vi "Turret.vi"(5 "turret":T1, 7 "top view":T1, 9 "angle":dbl, 11 "Refnum in":T1) -> (3 "Refnum out":T1)   [LabVIEW 2018]
uses:
  <vilib>/vision/Image Controls.llb/IMAQ Image.ctl
  <vilib>/vision/NI_Vision_Development_Module.lvlib
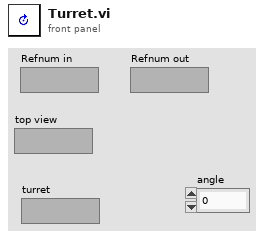
[diagram p1: front panel]
types:
  T1 = typedef "IMAQ Image.ctl" = refnum<image>
  T2 = cluster{"Blue or Luma":u8, "Green or Sat Plane":u8, "Red or Hue Plane":u8, "Alpha":u8}
  T3 = cluster{"Desired Font (Application)":enum16{"User-specified Font", "Application Font", "System Font", "Dialog Font"}, "[User-specified Font]":cluster{"Font Name":string, "Size":i16, "Strikeout?":bool, "Italic?":bool, "Underline?":bool, "Outline?":bool, "Shadow?":bool, "Bold?":bool, "Rotation Angle":dbl}, "Horizontal Alignment":i16, "Vertical Alignment":i16}
  T4 = typedef "Image Type" = u32
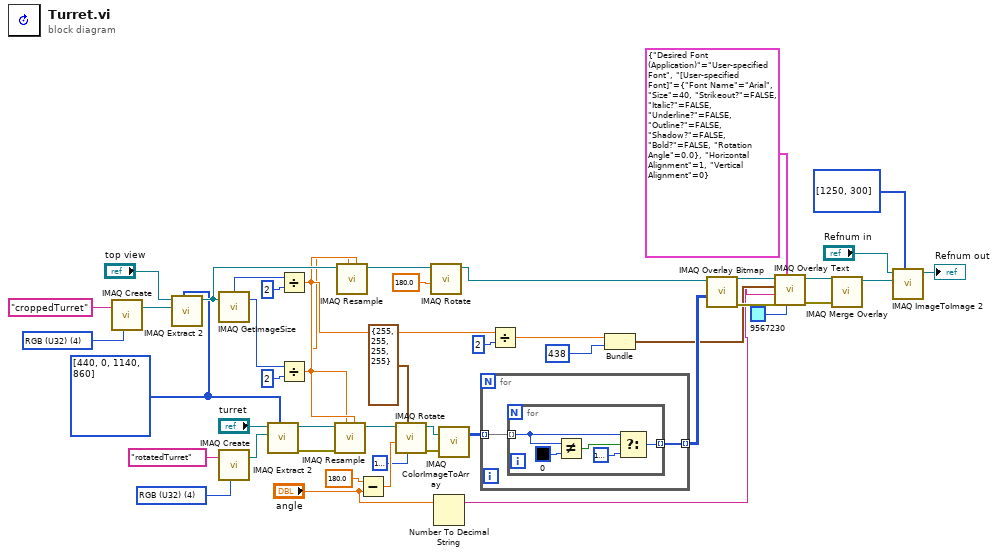
[diagram p0: block diagram]
diagram:
  w32 = T4 4 items=["Grayscale (U8)", "Grayscale (I16)", "Grayscale (SGL)", "Complex (CSG)", "RGB (U32)", "HSL (U32)", "RGB (U64)", "Grayscale (U16)"] ("Image Type")
  w40 = T4 4 items=["Grayscale (U8)", "Grayscale (I16)", "Grayscale (SGL)", "Complex (CSG)", "RGB (U32)", "HSL (U32)", "RGB (U64)", "Grayscale (U16)"] ("Image Type")
  w28 = i32[] [440, 0, 1140, 860] ("Optional Rectangle")
  n1 = call "IMAQ Create"("Image Name"="croppedTurret", "Image Type"=w40) -> ("New Image"=w41:T1)  [unwired: 3 in, 1 out]
  n2 = call "IMAQ Extract 2"("Optional Rectangle"=w28, "Image Dst"=w41, "Image Src"="top view") -> ("Image Dst Out"=w39:T1)  [unwired: 7 in, 1 out]
  n3 = call "IMAQ GetImageSize"("Image"=w39) -> ("Y Resolution"=w38:i32, "X Resolution"=w37:i32)  [unwired: 3 in, 1 out]
  n4 = call "IMAQ Create"("Image Name"="rotatedTurret", "Image Type"=w32) -> ("New Image"=w30:T1)  [unwired: 3 in, 1 out]
  n5 = call "IMAQ Extract 2"("Optional Rectangle"=w28, "Image Dst"=w30, "Image Src"="turret") -> ("error out"=w27:errorcluster, "Image Dst Out"=w26:T1)  [unwired: 7 in]
  n6 = Divide(x=w37, y=2) -> (x/y=w2:dbl)
  n7 = Divide(x=w38, y=2) -> (x/y=w1:dbl)
  n8 = call "IMAQ Resample"("X Resolution"=w2, "Y Resolution"=w1, "error in (no error)"=w27, "Image Src"=w26) -> ("Image Dst Out"=w25:T1)  [unwired: 6 in, 1 out]
  n9 = call "IMAQ Resample"("X Resolution"=w2, "Y Resolution"=w1, "Image Src"=w39) -> ("Image Dst Out"=w34:T1)  [unwired: 7 in, 1 out]
  n10 = Subtract(x=180.0 ("y"), y="angle") -> (x-y=w20:dbl)
  n11 = call "IMAQ Rotate"("Replace Value"=u32 16777216, "Color Replace Value"=T2 {"Blue or Luma"=255, "Green or Sat Plane"=255, "Red or Hue Plane"=255, "Alpha"=255}, "Angle (degrees)"=w20, "Image Src"=w25) -> ("error out"=w21:errorcluster, "Image Dst Out"=w22:T1)  [unwired: 6 in]
  n12 = call "IMAQ Rotate"("Angle (degrees)"=sgl 180.0, "Image Src"=w34) -> ("Image Dst Out"=w24:T1)  [unwired: 8 in, 1 out]
  n13 = Number To Decimal String(number="angle") -> (decimal integer string=w5:string)  [unwired: 1 in]
  n14 = call "IMAQ ColorImageToArray"("Image"=w22, "error in (no error)"=w21) -> ("Image Pixels (U32)"=w18:u32[][])  [unwired: 2 in, 2 out]
  n15 = for {
    tunnel: w18 -> [w48] mode=indexing
    tunnel: [w47] -> w17 mode=indexing
    n16 = for {
      tunnel: w48 -> [w51] mode=indexing
      tunnel: [w50] -> w47 mode=indexing
      n17 = Not Equal?(x=w51, y=u32 0) -> (x != y?=w52:bool)
      n18 = Select(t=w51, s=w52, f=u32 16777216) -> (s? t:f=w50:u32)
    }
  }
  n19 = Divide(x=w2, y=2) -> (x/y=w9:dbl)
  n20 = Bundle(w9, "y"=438) -> (w8:cluster{dbl, "y":i32})  [unwired: 1 in]
  n21 = call "IMAQ Overlay Bitmap"("Bitmap"=w17, "Image"=w24) -> ("error out"=w13:errorcluster, "Image Out"=w14:T1)  [unwired: 8 in]
  n22 = call "IMAQ Overlay Text"("Text Color (black)"=u32 9567230, "Font, Size & Style"=T3 {"Desired Font (Application)"=enum."User-specified Font", "[User-specified Font]"={"Font Name"="Arial", "Size"=40, "Strikeout?"=FALSE, "Italic?"=FALSE, "Underline?"=FALSE, "Outline?"=FALSE, "Shadow?"=FALSE, "Bold?"=FALSE, "Rotation Angle"=0.0}, "Horizontal Alignment"=1, "Vertical Alignment"=0}, "error in (no error)"=w13, "String"=w5, "Origin"=w8, "Image"=w14) -> ("error out"=w16:errorcluster, "Image Out"=w15:T1)  [unwired: 4 in]
  n23 = call "IMAQ Merge Overlay"("error in (no error)"=w16, "Image Src"=w15) -> ("Image Dst Out"=w23:T1)  [unwired: 8 in, 1 out]
  n24 = call "IMAQ ImageToImage 2"("Offset Left/Top"=i32[] [1250, 300], "Image Src (Small)"=w23, "Image Src (Large)"="Refnum in") -> ("Image Dst Out"=→"Refnum out":T1)  [unwired: 7 in, 1 out]
